vi "HapticSTM_nano.vi"() -> ()   [LabVIEW 2019]
uses:
  <vilib>/sound2/lvsound2.llb/Sampling Mode.ctl
  <vilib>/sound2/lvsound2.llb/Sound Data Format.ctl
  SubVIs/GlobalClicksHeight_nano.vi
  <vilib>/sound2/lvsound2.llb/Sound Output Set Volume (Single).vi
  <vilib>/sound2/lvsound2.llb/Sound Output Write (DBL Single).vi
  <vilib>/Utility/file.llb/Read Delimited Spreadsheet (DBL).vi
  Feedbackless - TestData/SubVIs/GlobalClicksHeight_flt.vi
  Program Files/National Instruments/LabVIEW 2019/user.lib/HapticSTM/HapticSTM.lvlib
  <vilib>/ptbypt/NI_PtbyPt.lvlib
  <userlib>/Nanonis Prog Interface V5/Nanonis Prog Interface.lvlib
panel:
  in  "Version?":bool=TRUE
  in  "Setpoint (pA)":dbl=100.0
  in  "Depth (pA)":dbl=280.0
  in  "Tab Control":T1(tab)
  out "ms/loop":u32=30
  in  "Z Write?":bool
  in  "Sound\nActivation":bool=TRUE
  in  "Sensitivity":dbl=1.0 format="%.1f"
  in  "Volume":dbl(slide)=50.0 scale=0.0..100.0
  in  "Device ID":u32
  out "function return":i32
  in  "Surface Shift (in)":dbl format="%.1f"
  in  "Scaling?":bool
  out "Setpoint (pA)":dbl
  in  "Maximum (pA)":dbl=7000.0
  out "Filtered Current (pA)":dbl format="%.1f"
  out "Current (pA)":dbl format="%.1f"
  out "Oy":dbl
  out "Ox":dbl
  out "W":dbl
  out "H":dbl
  out "Z Write":dbl format="%^.1e"
  out "Z Read":dbl format="%^#.1e"
  in  "Planing?":bool
  out "Button":bool
  out "Fy":dbl format="%.1f"
  out "Fz":dbl format="%.1f"
  out "Fx":dbl format="%.1f"
  out "x":dbl format="%.1f"
  out "y":dbl format="%.1f"
  out "z":dbl format="%0.1f"
  in  "Mode":u16(ring) items=["Log w/ Exp Z", "Log w/ Lin Z"]
  in  "Hardness":dbl=0.7 format="%.1f"
  in  "Reset Clicks":bool
  out "Clicks":i32
  in  "STOP":bool
  in  "START":bool
  out "Seq":i32
  out "SeqString":string
  out "Raw and Scaled Z Positions":cluster{dbl, "Y":dbl}(graph)
  out "Scaled Force and Current":T2(graph)
  # "Super Ultra Mega Haptic STM Controller 3000"
  # "Haptic Pen"
  # "Nanonis"
  # "Position"
  # "Force"
  # "Frame"
  # "Surface"
  # "Options"
  # "Addons"
  # "Test Data"
  # "Live"
  # "Sound Module"
  # "Small"
  # "Large"
  # "Current"
  # "Z Controller"
  # "No"
  # "Yes"
  # "Planing"
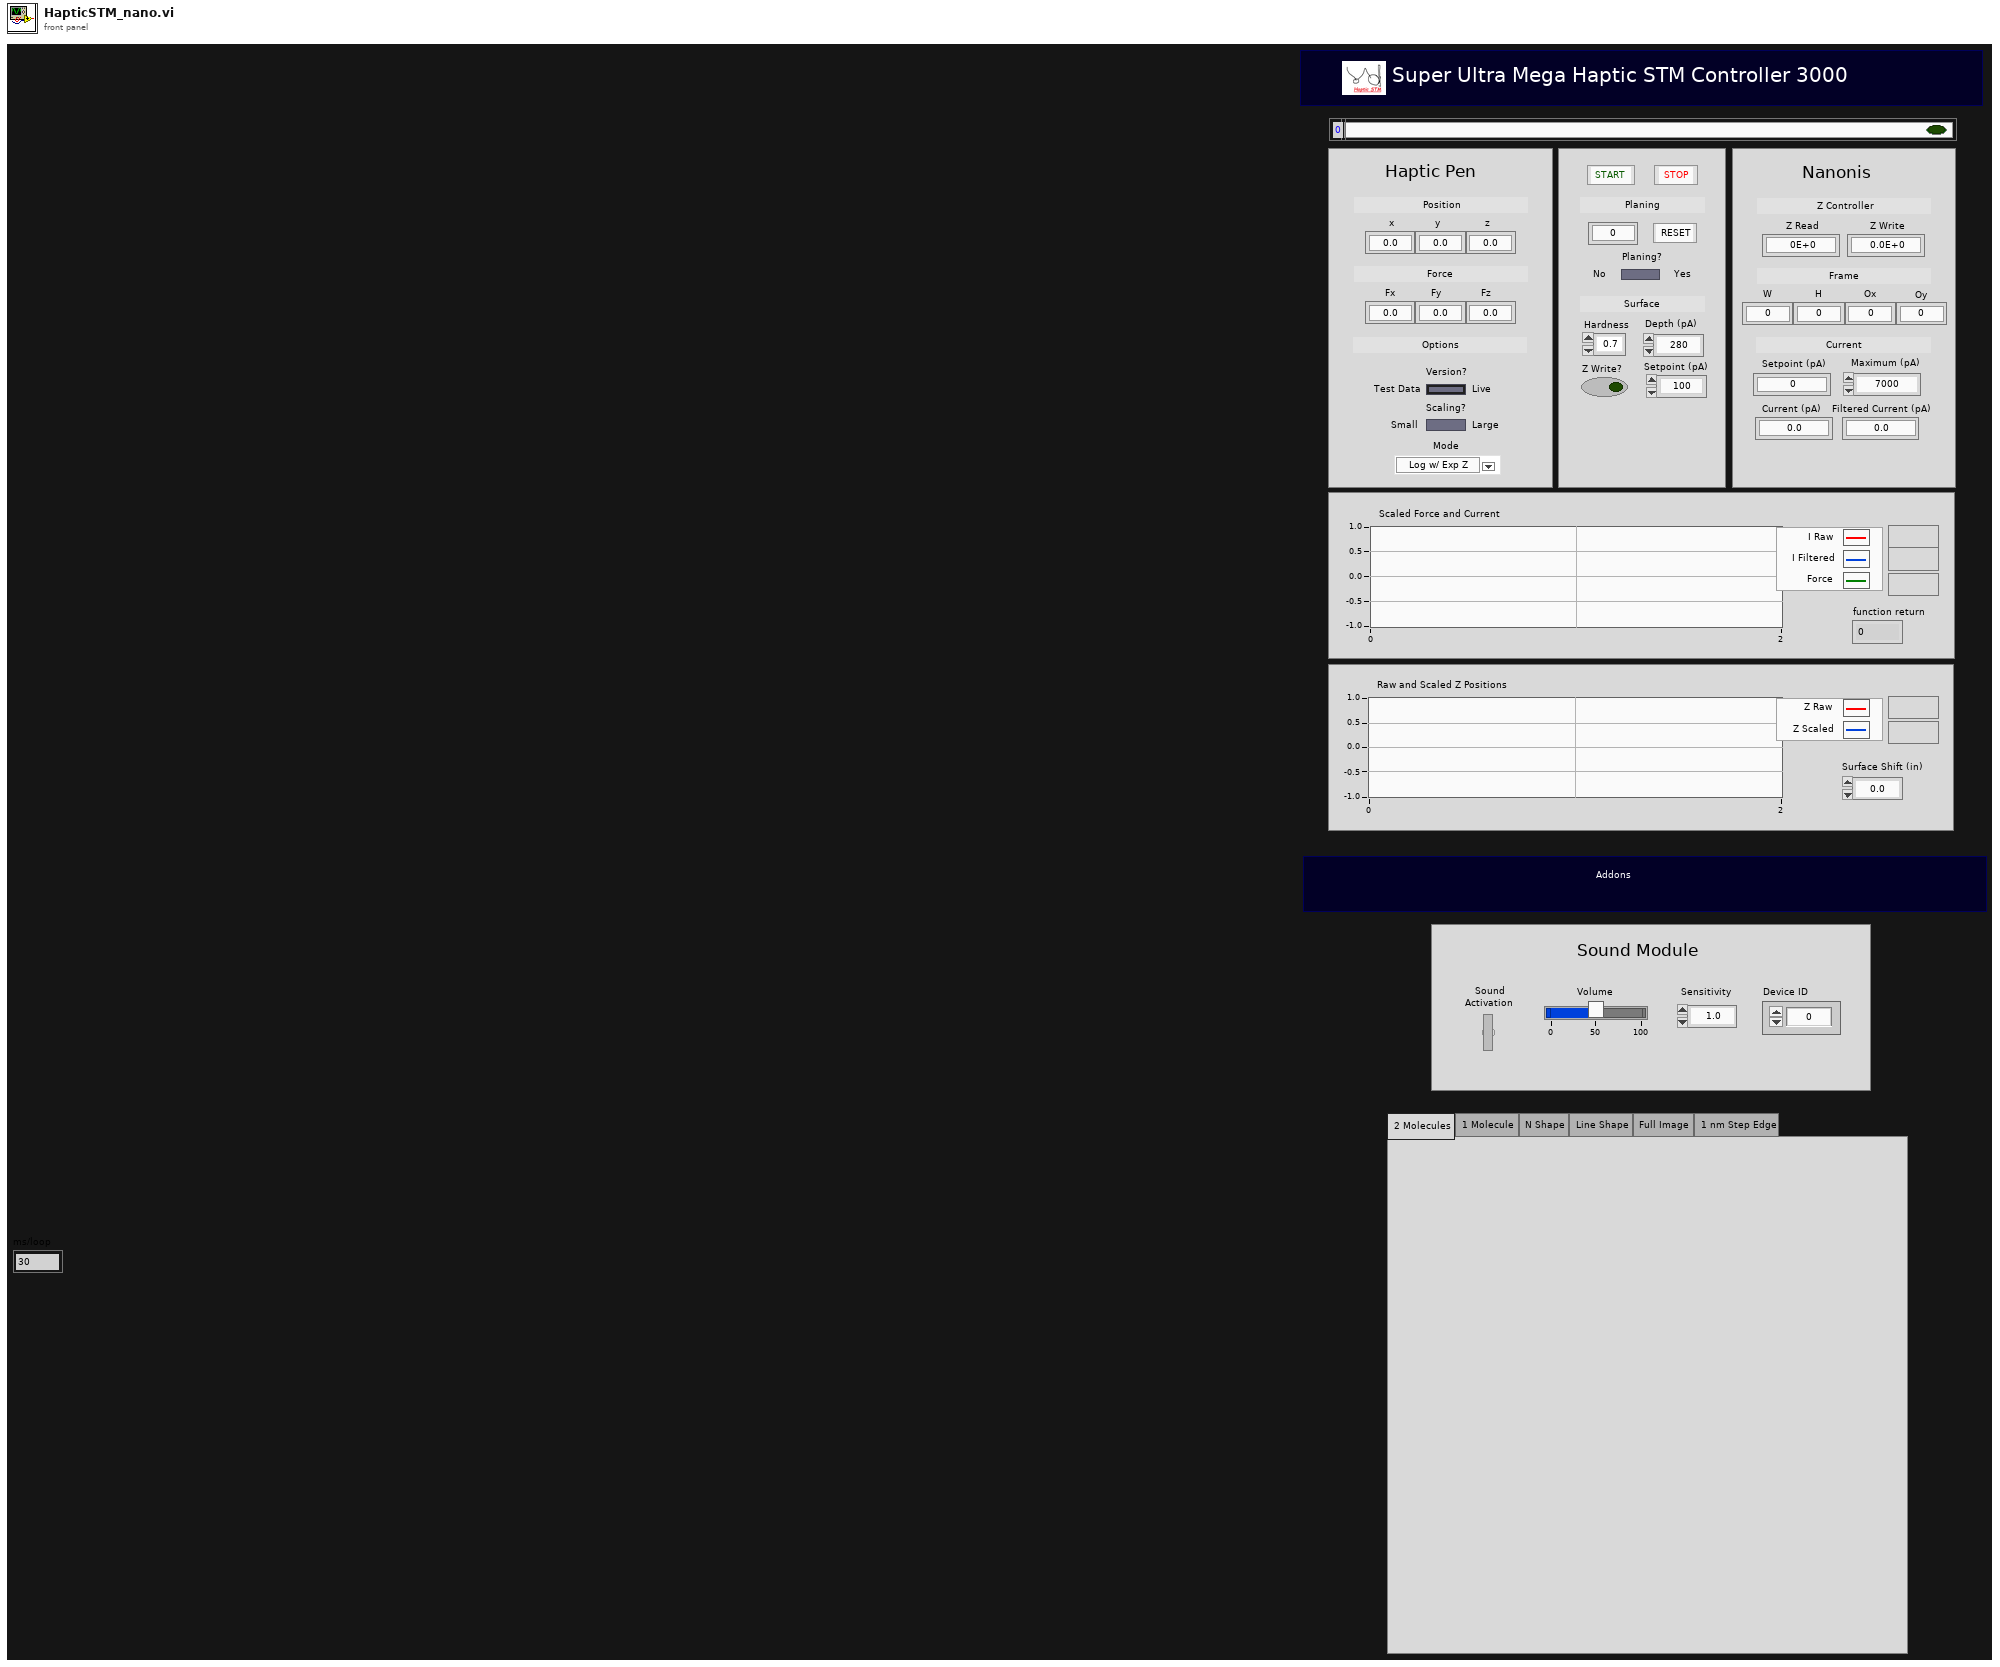
[diagram p1: front panel]
types:
  T1 = enum32{"2 Molecules", "1 Molecule", "N Shape", "Line Shape", "Full Image", "1 nm Step Edge"}
  T2 = cluster{"Current (pA)":dbl, "Filtered Current (pA)":dbl, dbl}
  T3 = typedef "Sound Data Format.ctl" = cluster{"sample rate (S/s)":dbl, "number of channels":i32, "bits per sample":i32}
  T4 = typedef "Sampling Mode.ctl" = i32
  T5 = cluster{"Size (m)":cluster{"Width":sgl, "Height":sgl}, "Center coordinates (m)":cluster{"Xc":sgl, "Yc":sgl}}
  T6 = typedef "Sound Output Task ID.ctl" = u32
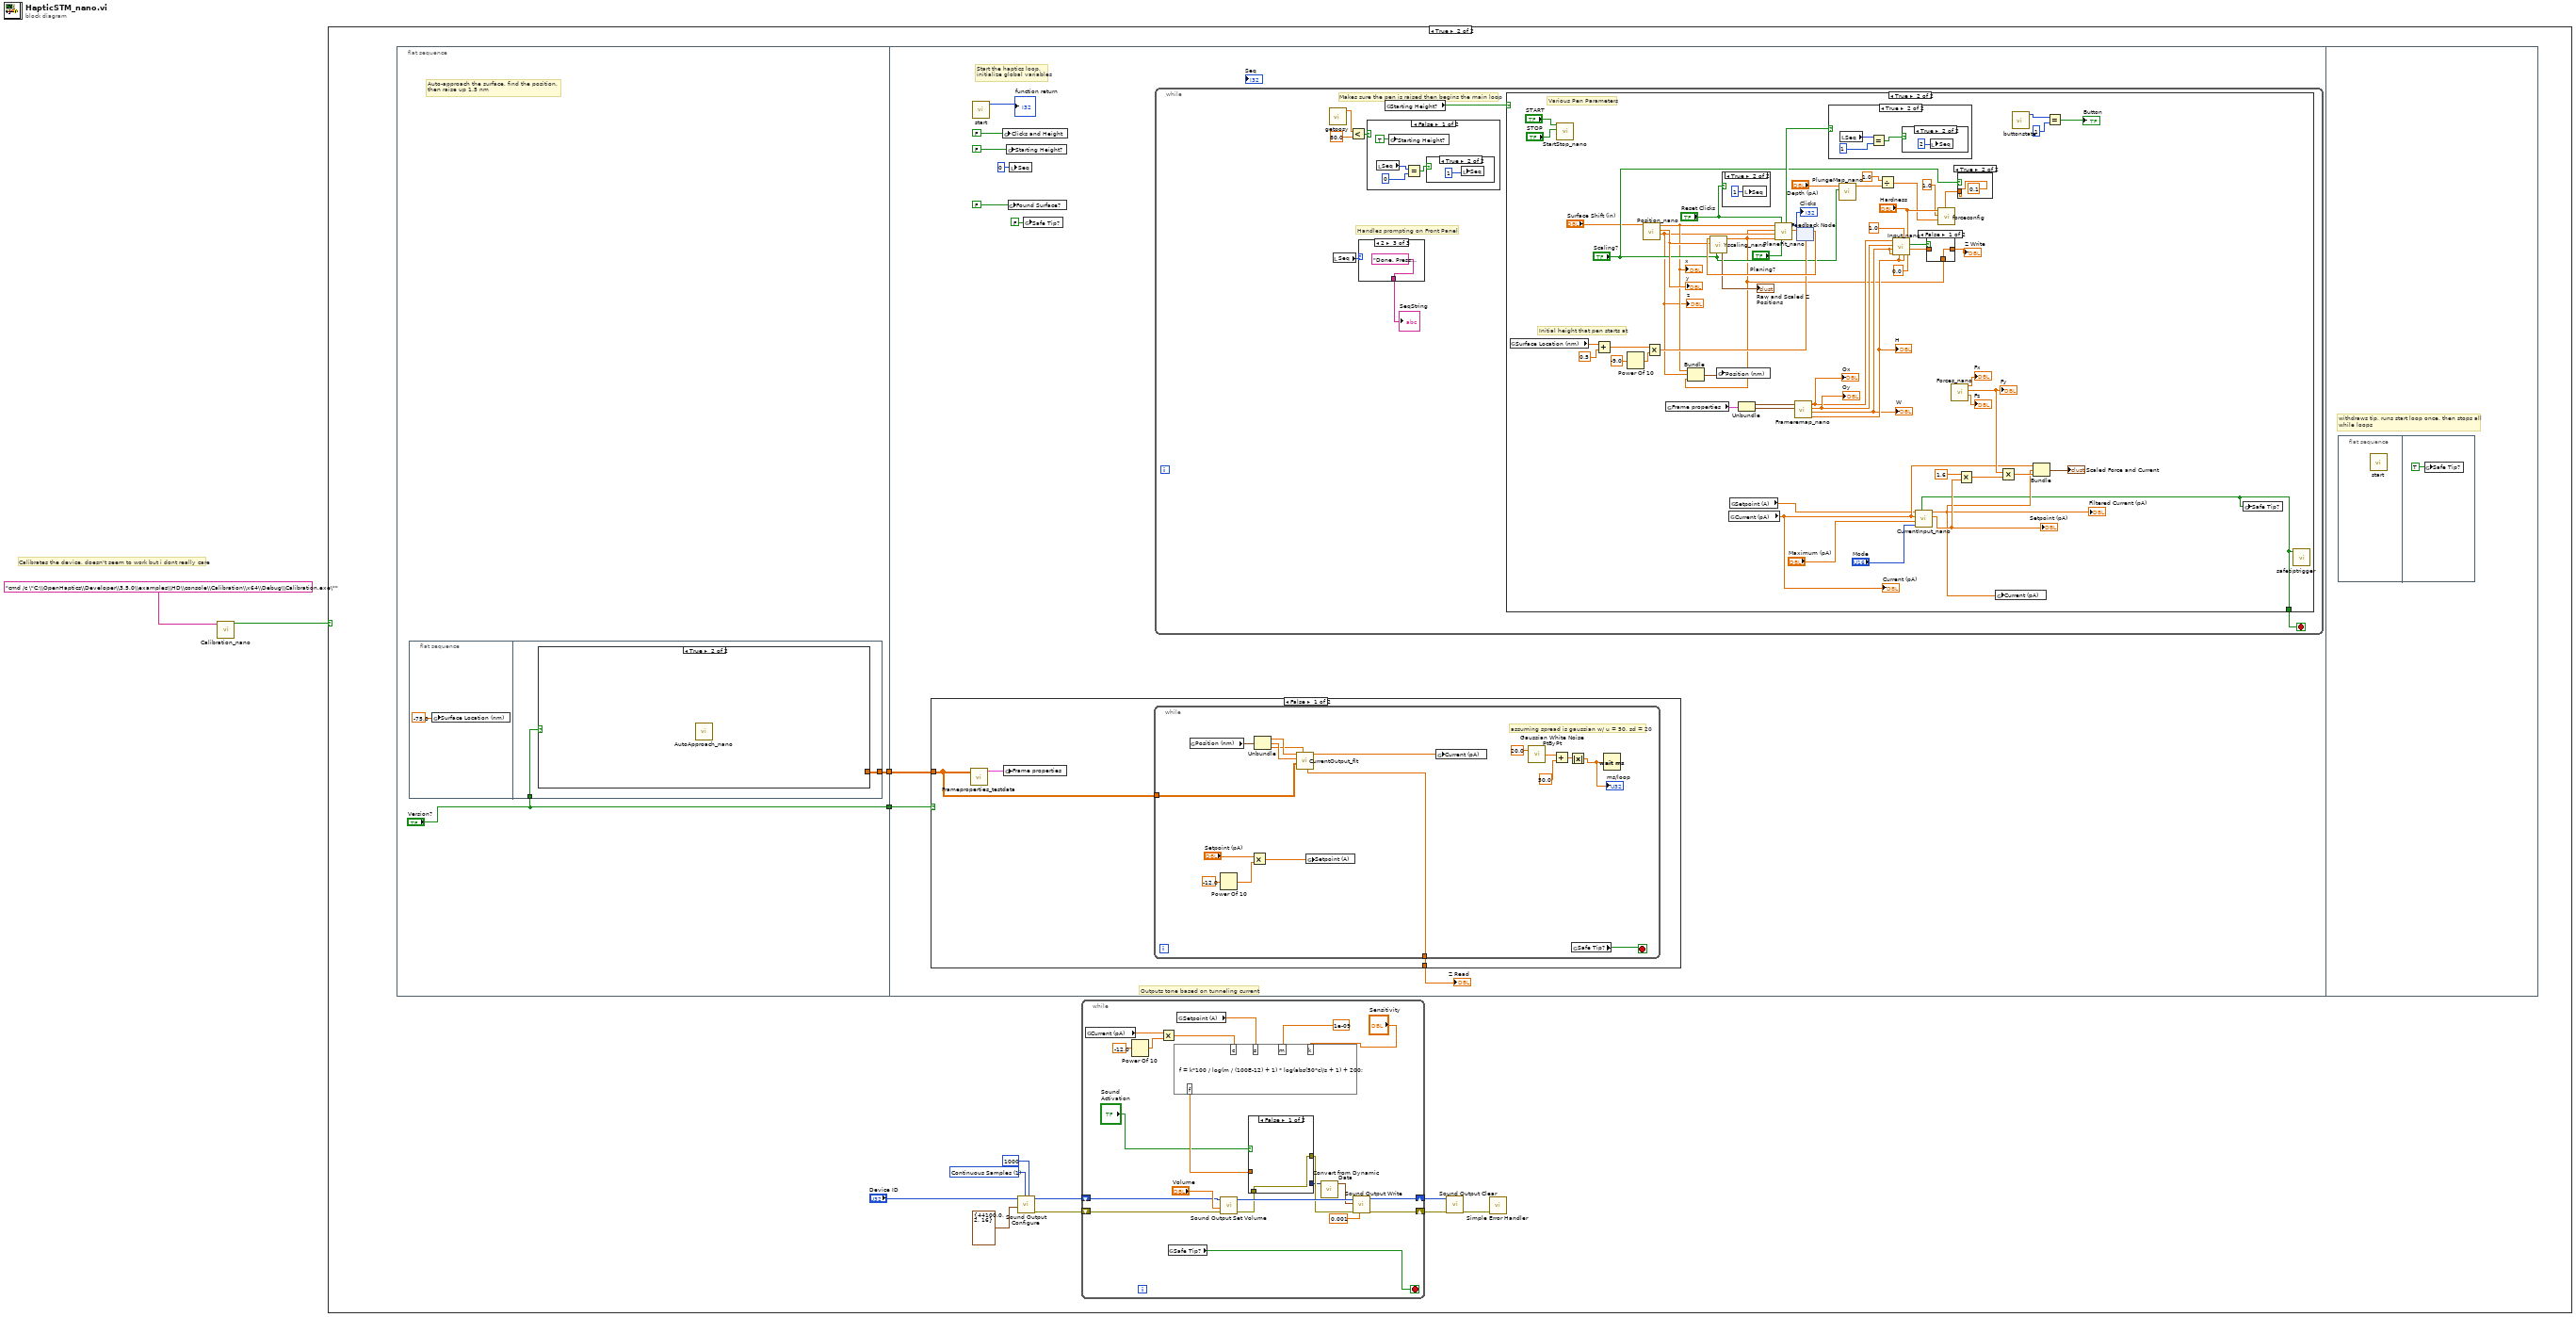
[diagram p0: block diagram]
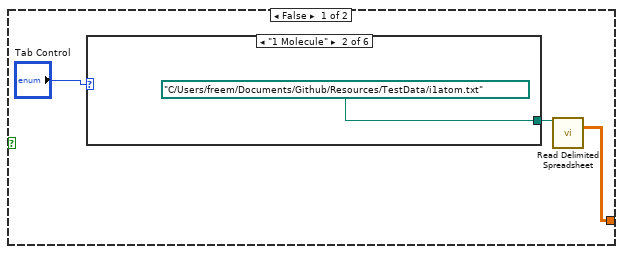
[diagram p3: hidden frame]
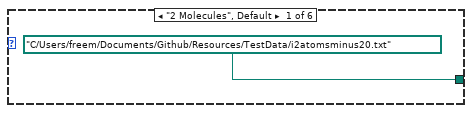
[diagram p4: hidden frame]
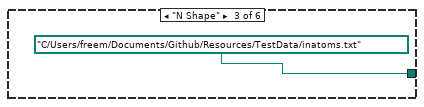
[diagram p5: hidden frame]
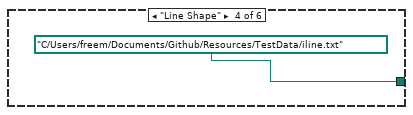
[diagram p6: hidden frame]
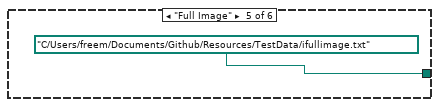
[diagram p7: hidden frame]
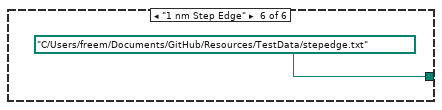
[diagram p8: hidden frame]
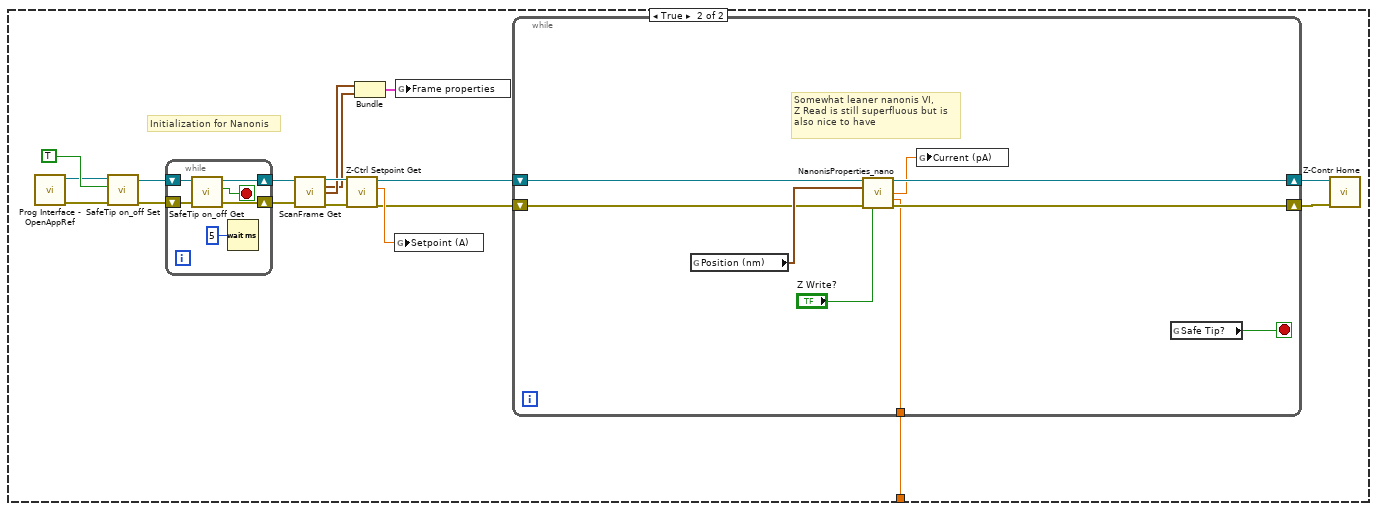
[diagram p9: hidden frame]
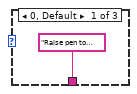
[diagram p10: hidden frame]
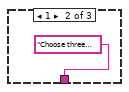
[diagram p11: hidden frame]
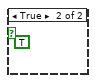
[diagram p13: hidden frame]
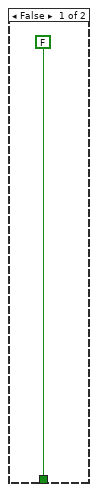
[diagram p14: hidden frame]
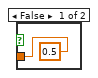
[diagram p15: hidden frame]
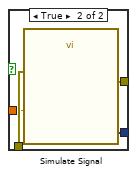
[diagram p20: hidden frame]
diagram:
  # "Calibrates the device, doesn't seem to work but i dont really care"
  n1 = call "Calibration_nano.vi"("command line"="cmd /c \"C:\\OpenHaptics\\Developer\\3.5.0\\examples\\HD\\console\\Calibration\\x64\\Debug\\Calibration.exe\"") -> ("Calibration Complete?"=w2:bool)  [unwired: 10 in]
  n2 = case shown="True" w2 {
    frame False {
    }
    frame True {
      w12 = T4 1 items=["Finite Samples", "Continuous Samples"] ("sample mode")
      # "Outputs tone based on tunneling current"
      n3 = flat-sequence {
        tunnel: ["Version?"] -> w4
        tunnel: [w14] -> w3
        tunnel: w4 -> [w29]
        tunnel: w3 -> [w28]
        frame #0 {
          # "Auto-approach the surface, find the position, \nthen raise up 1.5 nm"
          n4 = flat-sequence {
            tunnel: "Version?" -> [w18]
            tunnel: [w17] -> w14
            frame #0 {
              n5 = global write "GlobalClicksHeight_nano.vi" "Surface Location (nm)"(-75.0 ("Surface Location")) -> ()
            }
            frame #1 {
              n6 = case shown="True" w18 {
                tunnel: [w20 _] -> w17
                frame False {
                  n7 = case shown="\"1 Molecule\"" "Tab Control" {
                    tunnel: [path "C:/Users/freem/Documents/Github/Resources/TestData/i2atomsminus20.txt" ("file path (dialog if empty)") path "C:/Users/freem/Documents/Github/Resources/TestData/i1atom.txt" ("file path (dialog if empty)") path "C:/Users/freem/Documents/Github/Resources/TestData/inatoms.txt" ("file path (dialog if empty)") path "C:/Users/freem/Documents/Github/Resources/TestData/iline.txt" ("file path (dialog if empty)") path "C:/Users/freem/Documents/Github/Resources/TestData/ifullimage.txt" ("file path (dialog if empty)") path "C:/Users/freem/Documents/GitHub/Resources/TestData/stepedge.txt" ("file path (dialog if empty)")] -> w21
                    frame "2 Molecules", Default {
                    }
                    frame "1 Molecule" {
                    }
                    frame "N Shape" {
                    }
                    frame "Line Shape" {
                    }
                    frame "Full Image" {
                    }
                    frame "1 nm Step Edge" {
                    }
                  }
                  n8 = call-poly <vilib>:"Read Delimited Spreadsheet.vi"("file path (dialog if empty)"=w21) -> ("all rows"=w20:dbl[][])  [unwired: 9 in, 5 out]
                }
                frame True {
                  n9 = call "AutoApproach_nano.vi"() -> ()  [unwired: 12 in]
                }
              }
            }
          }
        }
        frame #1 {
          # "Start the haptics loop,\ninitialize global variables"
          n10 = case shown="False" w29 {
            tunnel: [w39 w60] -> w30
            tunnel: w28 -> [w38 _]
            frame False {
              n11 = call "Frameproperties_testdata.vi"("array"=w38) -> ("Frame properties"=w37:cluster{cluster{dbl, dbl}, cluster{dbl, dbl}})  [unwired: 10 in]
              n12 = global write "GlobalClicksHeight_nano.vi" "Frame properties"(w37) -> ()
              n13 = while {
                tunnel: [w46] -> w39
                tunnel: w38 -> [w44]
                stop <- w56 stop-if-true
                # "assuming spread is gaussian w/ u = 50, sd = 20"
                n14 = global read "GlobalClicksHeight_nano.vi" "Position (nm)"() -> (w45:cluster{"X":dbl, "Z":dbl, "Y":dbl})
                n15 = Power Of 10(x=-12.0) -> (10^x=w42:dbl)
                n16 = Multiply(x="Setpoint (pA)", y=w42) -> (x*y=w40:dbl)
                n17 = Unbundle(w45) -> ("X"=w55:dbl, "Z"=w54:dbl, "Y"=w52:dbl)
                n18 = call "CurrentOutput_flt.vi"("y scaled"=w52, "array"=w44, "Z Input"=w54, "X Input"=w55) -> ("Current Out (pA)"=w53:dbl, "Zread"=w46:dbl)  [unwired: 6 in]
                n19 = global write "GlobalClicksHeight_nano.vi" "Setpoint (A)"(w40) -> ()
                n20 = global write "GlobalClicksHeight_flt.vi" "Current (pA)"(w53) -> ()
                n21 = call <vilib>:"Gaussian White Noise PtByPt.vi"("standard deviation"=20.0) -> ("Gaussian white noise"=w50:dbl)  [unwired: 2 in]
                n22 = Add(x=w50, y=50.0) -> (x+y=w48:dbl)
                n23 = Absolute Value(x=w48) -> (abs(x)=w47:dbl)
                "ms/loop" <- w47
                n24 = global read "GlobalClicksHeight_flt.vi" "Safe Tip?"() -> (w56:bool)
                n25 = Wait (ms)(milliseconds to wait=w47) -> ()  [unwired: 1 out]
              }
            }
            frame True {
              # "Initialization for Nanonis"
              n26 = call <userlib>:"Prog Interface - OpenAppRef.vi"() -> ("Error out"=w72:errorcluster, "Application reference"=w73:refnum<vi>)  [unwired: 6 in]
              n27 = call <userlib>:"SafeTip on_off Set.vi"("error in (no error)"=w72, "SafeTip ON/OFF"=TRUE, "Application ref in"=w73) -> ("error out"=w70:errorcluster, "Application ref out"=w71:refnum<vi>)  [unwired: 7 in]
              n28 = while {
                shift-right: [w77] -> w69
                shift-left: w71 -> [w79]
                shift-right: [w76] -> w68
                shift-left: w70 -> [w78]
                stop <- w80 stop-if-true
                n29 = call <userlib>:"SafeTip on_off Get.vi"("error in (no error)"=w78, "Application ref in"=w79) -> ("error out"=w76:errorcluster, "SafeTip on/off status"=w80:bool, "Application ref out"=w77:refnum<vi>)  [unwired: 7 in]
                n30 = Wait (ms)(milliseconds to wait=u32 5) -> ()  [unwired: 1 out]
              }
              n31 = call <userlib>:"ScanFrame Get.vi"("Application ref in"=w69, "error in (no error)"=w68) -> ("Application ref out"=w67:refnum<vi>, "Center coordinates (m)"=w57:cluster{"Xc":sgl, "Yc":sgl}, "Size (m)"=w58:cluster{"Width":sgl, "Height":sgl}, "error out"=w66:errorcluster)  [unwired: 9 in, 1 out]
              n32 = call <userlib>:"Z-Ctrl Setpoint Get.vi"("error in (no error)"=w66, "Application ref in"=w67) -> ("error out"=w63:errorcluster, "Z Controller setpoint"=w65:sgl, "Application ref out"=w64:refnum<vi>)  [unwired: 6 in]
              n33 = Bundle("Size (m)"=w58, "Center coordinates (m)"=w57) -> (w59:T5)  [unwired: 1 in]
              n34 = global write "GlobalClicksHeight_nano.vi" "Setpoint (A)"(w65) -> ()
              n35 = global write "GlobalClicksHeight_nano.vi" "Frame properties"(w59) -> ()
              n36 = while {
                shift-right: [w83] -> w61
                shift-left: w63 -> [w85]
                shift-right: [w84] -> w62
                shift-left: w64 -> [w87]
                tunnel: [w81] -> w60
                stop <- w89 stop-if-true
                # "Somewhat leaner nanonis VI, \nZ Read is still superfluous but is\nalso nice to have"
                n37 = global read "GlobalClicksHeight_nano.vi" "Position (nm)"() -> (w88:cluster{"X":dbl, "Z":dbl, "Y":dbl})
                n38 = call "NanonisProperties_nano.vi"("Application ref in"=w87, "Position (nm)"=w88, "error in (no error)"=w85, "Z Write?"="Z Write?") -> ("Application ref out"=w84:refnum<vi>, "Current (pA)"=w82:sgl, "Z Read (m)"=w81:sgl, "error out"=w83:errorcluster)  [unwired: 8 in]
                n39 = global write "GlobalClicksHeight_nano.vi" "Current (pA)"(w82) -> ()
                n40 = global read "GlobalClicksHeight_nano.vi" "Safe Tip?"() -> (w89:bool)
              }
              n41 = call <userlib>:"Z-Contr Home.vi"("Error in (no error)"=w61, "Application ref in"=w62) -> ()  [unwired: 8 in, 2 out]
            }
          }
          "Z Read" <- w30
          n42 = call "start.vi"() -> ("function return"=→"function return":i32)  [unwired: 11 in]
          n43 = global write "GlobalClicksHeight_nano.vi" "Clicks and Height"(FALSE ("Clicks and Height")) -> ()
          n44 = global write "GlobalClicksHeight_nano.vi" "Starting Height?"(FALSE ("Clicks and Height")) -> ()
          n45 = global write "GlobalClicksHeight_nano.vi" "Found Surface?"(FALSE ("Clicks and Height")) -> ()
          n46 = local write "Seq"(0 ("Seq")) -> ()
          n47 = global write "GlobalClicksHeight_nano.vi" "Safe Tip?"(FALSE ("Safe Tip?")) -> ()
          n48 = while {
            stop <- w90 stop-if-true
            # "Makes sure the pen is raised then begins the main loop"
            # "Handles prompting on Front Panel"
            n49 = call "getposy.vi"() -> ("function return"=w96:dbl)  [unwired: 11 in]
            n50 = local read "Seq"() -> (w92:i32)
            n51 = Less?(x=w96, y=80.0) -> (x < y?=w94:bool)
            n52 = case shown="2" w92 {
              tunnel: ["Raise pen to begin." "Choose three points, then raise the arm to plane." "Done. Press 'STOP' to stop at anytime."] -> w91
              frame 0, Default {
              }
              frame 1 {
              }
              frame 2 {
              }
            }
            "SeqString" <- w91
            n53 = case shown="False" w94 {
              frame False {
                n54 = local read "Seq"() -> (w102:i32)
                n55 = global write "GlobalClicksHeight_nano.vi" "Starting Height?"(TRUE ("Starting Height?")) -> ()
                n56 = Equal?(x=w102, y=0) -> (x = y?=w100:bool)
                n57 = case shown="True" w100 {
                  frame False {
                  }
                  frame True {
                    n58 = local write "Seq"(1 ("Seq")) -> ()
                  }
                }
              }
              frame True {
                (unwired) TRUE ("Clicks and Height")
              }
            }
            n59 = global read "GlobalClicksHeight_nano.vi" "Starting Height?"() -> (w93:bool)
            n60 = case shown="True" w93 {
              tunnel: [FALSE ("Current Maxed?") w109] -> w90
              frame False {
              }
              frame True {
                # "Initial height that pen starts at"
                # "Various Pen Parameters"
                n61 = global read "GlobalClicksHeight_nano.vi" "Surface Location (nm)"() -> (w125:dbl)
                n62 = call "StartStop_nano.vi"("STOP"="STOP", "START"="START") -> ()  [unwired: 10 in]
                n63 = Add(x=w125, y=0.5) -> (x+y=w122:dbl)
                n64 = Power Of 10(x=-9.0) -> (10^x=w121:dbl)
                n65 = call "Position_nano.vi"("Shift"="Surface Shift (in)") -> ("Z"=w113:dbl, "Y"=w151:dbl, "X"=w114:dbl)  [unwired: 8 in]
                "x" <- w114
                "y" <- w151
                "z" <- w113
                n66 = Multiply(x=w122, y=w121) -> (x*y=w123:dbl)
                n67 = global read "GlobalClicksHeight_nano.vi" "Frame properties"() -> (w108:cluster{cluster{dbl, dbl}, cluster{dbl, dbl}})
                n68 = case shown="True" "Reset Clicks" {
                  frame False {
                  }
                  frame True {
                    n69 = local write "Seq"(1 ("Seq")) -> ()
                  }
                }
                n70 = global read "GlobalClicksHeight_nano.vi" "Current (pA)"() -> (w111:dbl)
                "Current (pA)" <- w111
                n71 = global read "GlobalClicksHeight_nano.vi" "Setpoint (A)"() -> (w110:dbl)
                n72 = Unbundle(w108) -> (w107:cluster{dbl, dbl}, w106:cluster{dbl, dbl})
                n73 = call "Frameremap_nano.vi"("Frame Origin (m)"=w106, "Frame Size (m)"=w107) -> ("FH (nm)"=w135:dbl, "FW (nm)"=w134:dbl, "Z Origin (nm)"=w133:dbl, "X Origin (nm)"=w132:dbl)  [unwired: 6 in]
                "H" <- w135
                "W" <- w134
                "Ox" <- w132
                "Oy" <- w133
                n74 = feedback #1(w123) -> (w157:dbl)
                n75 = call "Yscaling_nano.vi"("Scaling?"="Scaling?", "Y"=w151, "Plane Height (m)"=w157) -> ("y scaled (m)"=w112:dbl, "Zpos Graph (nm)"=→"Raw and Scaled Z Positions":cluster{dbl, "function return":dbl})  [unwired: 7 in]
                n76 = Bundle("X"=w114, "Z"=w113, "y scaled (m)"=w112) -> (w115:cluster{"X":dbl, "Z":dbl, "y scaled (m)":dbl})  [unwired: 1 in]
                n77 = global write "GlobalClicksHeight_nano.vi" "Position (nm)"(w115) -> ()
                n78 = call "PlaneFit_nano.vi"("Planing y/n?"="Planing?", "Reset Clicks"="Reset Clicks", "Y PEN"=w112, "Z"=w113, "Nano Z"=w112, "X"=w114) -> ("Plane Height (m)"=w158:dbl, "Clicks"=→"Clicks":i32, "Planing Done?"=w144:bool)  [unwired: 3 in]
                n79 = feedback-in #1(w158) -> ()
                n80 = case shown="True" w144 {
                  frame False {
                  }
                  frame True {
                    n81 = local read "Seq"() -> (w171:i32)
                    n82 = Equal?(x=w171, y=1) -> (x = y?=w169:bool)
                    n83 = case shown="True" w169 {
                      frame False {
                      }
                      frame True {
                        n84 = local write "Seq"(2 ("Seq")) -> ()
                      }
                    }
                  }
                }
                n85 = call "PlungeMap_nano.vi"("Scaling?"="Scaling?", "Input (pA)"="Depth (pA)") -> ("output"=w126:dbl)  [unwired: 9 in]
                n86 = Divide(x=1.0, y=w126) -> (x/y=w136:dbl)
                n87 = call "Input_nano.vi"("Current * 10^input"=0.0, "Sensitivity"="Hardness", "Scopez"=w135, "Drag"=1.0, "FH"=w135, "FW"=w134, "Scopex"=w134, "Z origin"=w133, "X origin"=w132) -> ("Scaled Current"=w138:dbl, "feedback"=w140:bool)  [unwired: 1 in]
                n88 = call "CurrentInput_nano.vi"("Mode"="Mode", "Maximum (pA)"="Maximum (pA)", "Current (pA)"=w111, "Setpoint (A)"=w110) -> ("Setpoint (pA)"=w128:dbl, "Filtered Current (pA)"=w119:dbl, "Safetip?"=w109:bool)  [unwired: 5 in]
                "Filtered Current (pA)" <- w119
                "Setpoint (pA)" <- w128
                n89 = case shown="False" w140 {
                  tunnel: [w166 w167] -> w139
                  tunnel: w138 -> [_ w167]
                  tunnel: w112 -> [w166 _]
                  frame False {
                  }
                  frame True {
                  }
                }
                "Z Write" <- w139
                n90 = call "Forces_nano.vi"() -> ("Fz"=→"Fz":dbl, "Fy"=w155:dbl, "Fx"=→"Fx":dbl)  [unwired: 9 in]
                "Fy" <- w155
                n91 = case shown="True" "Scaling?" {
                  tunnel: [0.5 0.1] -> w118
                  frame False {
                  }
                  frame True {
                  }
                }
                n92 = call "forceconfig.vi"("spc"=w118, "c"=w136, "b"=1.0, "a"="Hardness") -> ()  [unwired: 8 in]
                n93 = Multiply(x=1.6 ("y"), y=w128) -> (x*y=w152:dbl)
                n94 = global write "GlobalClicksHeight_nano.vi" "Current (pA)"(w119) -> ()
                n95 = Multiply(x=w155, y=w152) -> (x*y=w154:dbl)
                n96 = call "buttonstate.vi"() -> ("function return"=w150:i32)  [unwired: 11 in]
                n97 = Bundle("Current (pA)"=w111, "Filtered Current (pA)"=w119, w154) -> (→"Scaled Force and Current":T2)  [unwired: 1 in]
                n98 = Equal?(x=w150, y=1) -> (x = y?=→"Button":bool)
                n99 = global write "GlobalClicksHeight_nano.vi" "Safe Tip?"(w109) -> ()
                n100 = call "safetiptrigger.vi"("triggered"=w109) -> ()  [unwired: 11 in]
              }
            }
          }
        }
        frame #2 {
          # "withdraws tip, runs start loop once, then stops all\nwhile loops"
          n101 = flat-sequence {
            frame #0 {
              n102 = call "start.vi"() -> ()  [unwired: 11 in, 1 out]
            }
            frame #1 {
              n103 = global write "GlobalClicksHeight_nano.vi" "Safe Tip?"(TRUE ("Safe Tip?")) -> ()
            }
          }
        }
      }
      n104 = call <vilib>:"Sound Output Configure.vi"("number of samples/ch"=1000 ("Number of Samples/ch"), "sample mode"=w12, "sound format"=T3 {"sample rate (S/s)"=44100.0, "number of channels"=2, "bits per sample"=16} ("Sound Format"), "device ID"="Device ID") -> ("error out"=w8:errorcluster, "task ID"=w9:T6)  [unwired: 6 in]
      n105 = while {
        shift-right: [w186] -> w7
        shift-left: w9 -> [w188]
        shift-right: [w185] -> w6
        shift-left: w8 -> [w187]
        stop <- w175 stop-if-true
        n106 = global read "GlobalClicksHeight_nano.vi" "Current (pA)"() -> (w178:dbl)
        n107 = Power Of 10(x=-12.0) -> (10^x=w180:dbl)
        n108 = Multiply(x=w178, y=w180) -> (x*y=w177:dbl)
        n109 = global read "GlobalClicksHeight_nano.vi" "Safe Tip?"() -> (w175:bool)
        n110 = global read "GlobalClicksHeight_nano.vi" "Setpoint (A)"() -> (w182:dbl)
        n111 = formula code="f = k*100 / log(m / (100E-12) + 1) * log(abs(50*c)/s + 1) + 200;"("c"=w177, "m"=1e-09 ("input variable"), "s"=w182, "k"="Sensitivity") -> ("f"=w181:dbl)
        n112 = call-poly <vilib>:"Sound Output Set Volume.vi"("error in (no error)"=w187, "volume"="Volume", "task ID"=w188) -> ("error out"=w191:errorcluster, "task ID out"=w194:T6)  [unwired: 7 in]
        n113 = case shown="False" "Sound\nActivation" {
          tunnel: w191 -> [w195 w199]
          tunnel: [w195 w198] -> w190
          tunnel: [_ w197] -> w189
          tunnel: w181 -> [_ w196]
          frame False {
          }
          frame True {
            n114 = call "Simulate Signal"("Frequency"=w196, "error in (no error)"=w199) -> ("Sine"=w197:dynamicdata, "error out"=w198:errorcluster)  [unwired: 12 in]
          }
        }
        n115 = call "Convert from Dynamic Data"("Dynamic Data Type"=w189) -> ("Waveform"=w192:waveform(dbl))  [unwired: 3 in]
        n116 = call-poly <vilib>:"Sound Output Write.vi"("timeout (sec)"=0.001, "error in (no error)"=w190, "data"=w192, "task ID"=w194) -> ("error out"=w185:errorcluster, "task ID out"=w186:T6)  [unwired: 6 in]
      }
      n117 = call <vilib>:"Sound Output Clear.vi"("error in (no error)"=w6, "task ID"=w7) -> ("error out"=w11:errorcluster)  [unwired: 9 in]
      n118 = call <vilib>:"Simple Error Handler.vi"("error in (no error)"=w11) -> ()  [unwired: 4 in, 5 out]
    }
  }
